vi "FGV_FromExternalProcessesEvent.vi"(7 "Command":T1, 8 "error in (no error)":errorcluster) -> (0 "error out":errorcluster, 3 "From ExternalProcess Event":refnum<user-event>)   [LabVIEW 2011]
uses:
  EnumFgvEventCommand.ctl
  FromExternalProcessesEvent.ctl
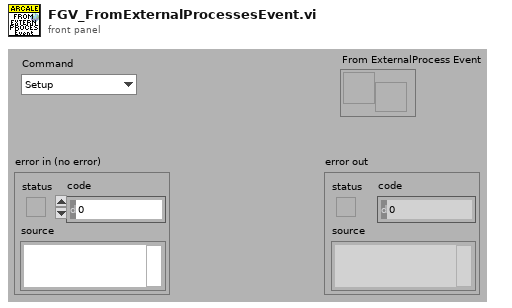
[diagram p1: front panel]
types:
  T1 = typedef "EnumFgvEventCommand.ctl" = enum16{"Setup", "Cleanup", "Get"}
  T2 = typedef "FromExternalProcessesEvent.ctl" = cluster{"vi reference":refnum<vi>, "variant":variant}
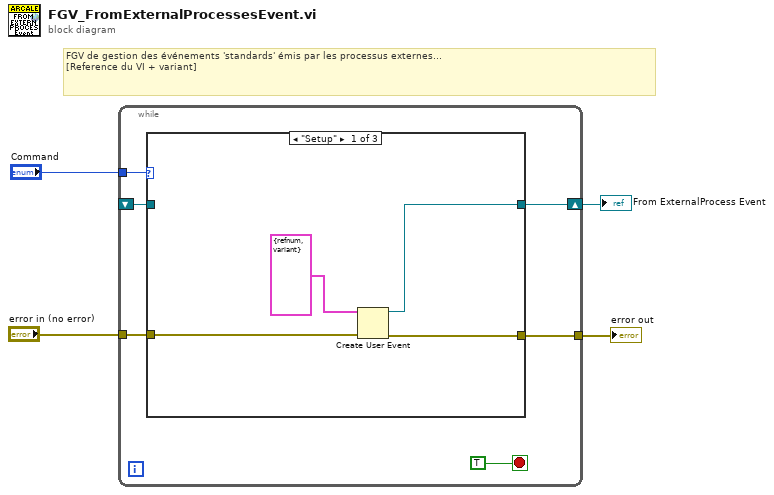
[diagram p0: block diagram]
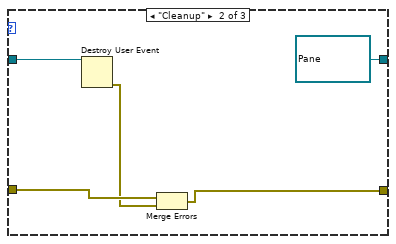
[diagram p2: hidden frame]
diagram:
  # "FGV de gestion des événements 'standards' émis par les processus externes...\n[Reference du VI + variant]"
  n1 = while {
    tunnel: "Command" -> [w9]
    tunnel: "error in (no error)" -> [w8]
    tunnel: [w7] -> w2
    shift-right: [w6] -> w1
    shift-left: _ -> [w5]
    stop <- TRUE stop-if-true
    n2 = case shown="\"Setup\"" w9 {
      tunnel: w8 -> [w14 w18 w20]
      tunnel: [w13 w16 w20] -> w7
      tunnel: [w12 refnum<user-event> refnum ("From Process Event") w21] -> w6
      tunnel: w5 -> [_ w19 w21]
      frame "Setup" {
        n3 = Create User Event(user event datatype=T2 {"vi reference"=refnum, "variant"=variant} ("From ExternalProcess Event"), error in=w14) -> (user event=w12:refnum<user-event>, error out=w13:errorcluster)
      }
      frame "Cleanup" {
        n4 = Destroy User Event(user event=w19) -> (error out=w17:errorcluster)  [unwired: 1 in]
        n5 = Merge Errors(w18, w17) -> (w16:errorcluster)
      }
      frame "Get" {
      }
    }
  }
  "error out" <- w2
  "From ExternalProcess Event" <- w1
